vi "L0.vi"(8 "error in (no error)":errorcluster) -> (0 "error out":errorcluster, 3 "function return":dbl)   [LabVIEW 2014, in "MASTTCSGET.lvlib"]
doc: "solar L0 coordinate(heliographic latitude longtitude)\n\n\n\n\n\n__declspec (dllexport) float L0();"
uses:
  MASTTCSGET.lvlib
  MASTTCSGET.dll
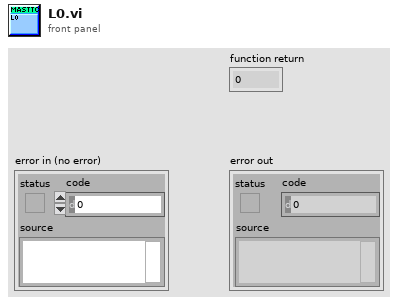
[diagram p1: front panel]
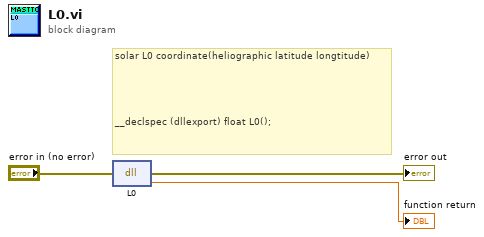
[diagram p0: block diagram]
diagram:
  # "solar L0 coordinate(heliographic latitude longtitude)\n\n\n\n\n\n__declspec (dllexport) float L0();"
  n1 = dll-call lib="F:/weekend/mast_controlsystem/MASTTCSGET.*" fn="L0"(error in="error in (no error)") -> (error out=→"error out":errorcluster, →"function return":dbl)  [unwired: 2 in, 1 out]
